vi "FieldDisplaySmall_OLD.vi"() -> ()   [LabVIEW 2025]
uses:
  <vilib>/Rock Robotics/WPI/ThirdParty/JAS_Junk/TrajLib/TypeDef/FieldDisp_ElementPicture.ctl
  <vilib>/Rock Robotics/WPI/ThirdParty/JAS_Junk/TrajLib/Rotation2d_CreateAngle.vi
  <vilib>/Rock Robotics/WPI/ThirdParty/JAS_Junk/TrajLib/Translation2d_Create.vi
  <vilib>/Rock Robotics/WPI/ThirdParty/JAS_Junk/TrajLib/VI/FieldDisp_Element_Rotate.vi
  <vilib>/Rock Robotics/WPI/ThirdParty/JAS_Junk/TrajLib/Conv_Meters_Inches.vi
  <vilib>/Rock Robotics/WPI/ThirdParty/JAS_Junk/TrajLib/Conv_Radians_Deg.vi
  <vilib>/picture/pixmap.llb/Flatten Pixmap.vi
  <vilib>/picture/pictutil.llb/Create Mask.vi
  <vilib>/picture/picture.llb/Draw Flattened Pixmap.vi
  <vilib>/Rock Robotics/WPI/ThirdParty/JAS_Junk/TrajLib/Trajectory_Library.lvlib
panel:
  out "Rear Side Last Sec Cnt":i32 format="%10.0f"
  out "Rear Back Last Sec Cnt":i32 format="%10.0f"
  out "Right Last Sec Cnt":i32 format="%10.0f"
  out "Left Last Sec Cnt":i32 format="%10.0f"
  out "ROBOT 2":T1
  out "Rear Side Tag Found":bool
  out "Rear Side Cam Conn":bool
  out "Rear Back Tag Found":bool
  out "Rear Back Cam Conn":bool
  out "Driver Orient Deg":dbl format="%11.1f"
  out "Driver Y Ft":dbl format="%11.2f"
  out "Driver X Ft":dbl format="%11.2f"
  out "ROBOT":T1
  out "Robot Orient Deg":dbl format="%11.1f"
  out "Robot Y Ft":dbl format="%11.2f"
  out "Robot X Ft":dbl format="%11.2f"
  out "Right April Tag Found":bool
  out "Left April Tag Found":bool
  out "Right Cam Connected":bool
  out "Left Cam Connected":bool
  out "Field Picture":picture
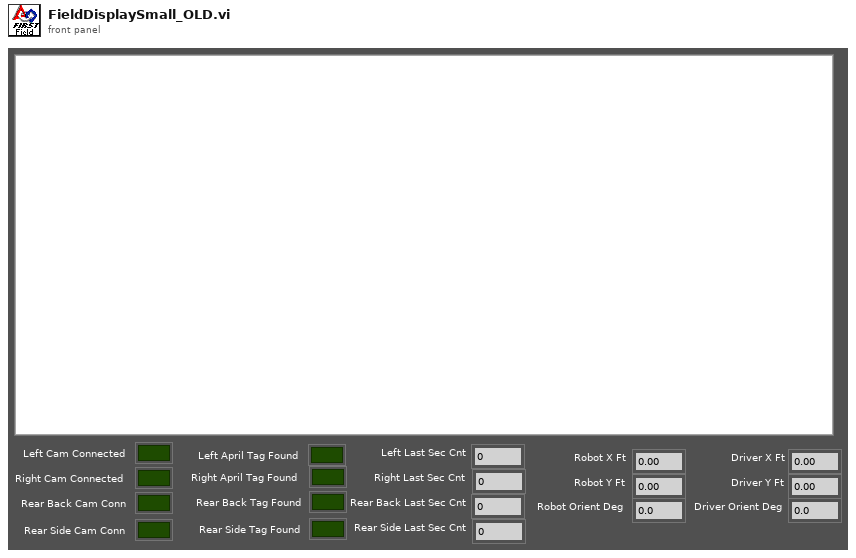
[diagram p1: front panel]
types:
  T1 = typedef "Trajectory_Library.lvlib/FieldDisp_ElementPicture.ctl" = picture
  T2 = typedef "Trajectory_Library.lvlib/FieldDisp_FieldElement.ctl" = cluster{"ONE-8-bit pixmap":u8[][], "Two-Array":cdb[][], "Three-Numeric":i32, "Four-Numeric":i32, "Five-Numeric":cdb, "Six-colors":u32[], "Seven-new element/subarray":u32, "Left Pixel":dbl, "Top Pixel":dbl, "Width Pix/Ft":dbl, "Height Pix/Ft":dbl, "Element Picture Ref":refnum<vi>}
  T3 = typedef "Trajectory_Library.lvlib/POSE2D.ctl" = cluster{"TRANSLATION":T4, "ROTATION":T5}
  T4 = typedef "Trajectory_Library.lvlib/TRANSLATION2D.ctl" = cluster{"X":dbl, "Y":dbl}
  T5 = typedef "Trajectory_Library.lvlib/ROTATION2D.ctl" = cluster{"VALUE":dbl, "COS":dbl, "SIN":dbl}
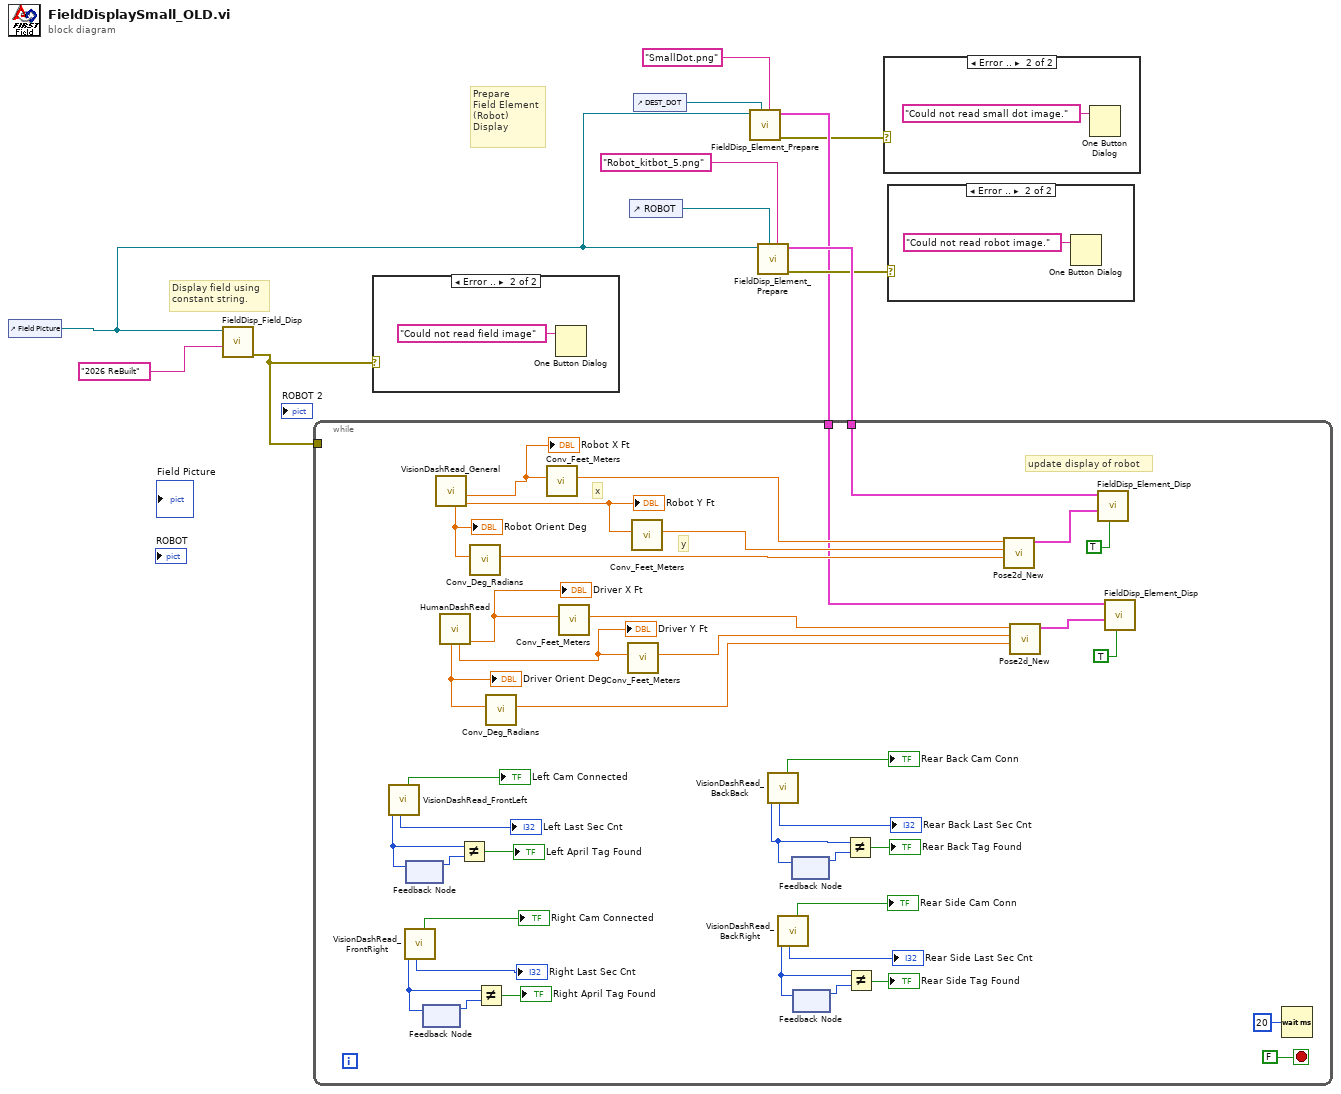
[diagram p0: block diagram]
diagram:
  # "Prepare\nField Element\n(Robot)\nDisplay"
  # "Display field using\nconstant string."
  n1 = control-ref of="Field Picture"() -> (w3:refnum<vi>)
  n2 = call <vilib>:"FieldDisp_Field_Disp.vi"("Field Selector"="2026 ReBuilt", "Picture in"=w3) -> ("error out"=w6:errorcluster)  [unwired: 9 in]
  n3 = case shown="Error .." w6 {
    frame No Error {
    }
    frame Error {
      n4 = One Button Dialog(message="Could not read field image") -> ()  [unwired: 1 in, 1 out]
    }
  }
  n5 = control-ref of="ROBOT"() -> (w9:refnum<vi>)
  n6 = control-ref of="DEST_DOT"() -> (w5:refnum<vi>)
  n7 = call <vilib>:"FieldDisp_Element_Prepare.vi"("Element File Name"="SmallDot.png" ("Picture FIle Name"), "Element Picture Ref"=w5, "Field Picture Ref"=w3) -> ("error out"=w1:errorcluster, "Field Element Info"=w2:T2)  [unwired: 7 in]
  n8 = call <vilib>:"FieldDisp_Element_Prepare.vi"("Element File Name"="Robot_kitbot_5.png" ("Picture FIle Name"), "Element Picture Ref"=w9, "Field Picture Ref"=w3) -> ("error out"=w7:errorcluster, "Field Element Info"=w8:T2)  [unwired: 7 in]
  n9 = while {
    tunnel: w8 -> [w51]
    tunnel: w6 -> [_]
    tunnel: w2 -> [w26]
    stop <- FALSE stop-if-true
    # "update display of robot"
    # "y"
    # "x"
    n10 = call "VisionDashRead_FrontLeft.vi"() -> ("FL Conn"=→"Left Cam Connected":bool, "FL Last Sec Cnt"=→"Left Last Sec Cnt":i64, "FL Count"=w36:i64)  [unwired: 2 in, 7 out]
    n11 = call "VisionDashRead_FrontRight.vi"() -> ("FR Conn"=→"Right Cam Connected":bool, "FR Last Sec Cnt"=→"Right Last Sec Cnt":i64, "FR Count"=w34:i64)  [unwired: 2 in, 7 out]
    n12 = feedback #1() -> (w47:i64)  [unwired: 1 in]
    n13 = feedback-in #1(w36) -> ()
    n14 = feedback #2() -> (w46:i64)  [unwired: 1 in]
    n15 = feedback-in #2(w34) -> ()
    n16 = call "VisionDashRead_General.vi"() -> ("PosYFt"=w39:dbl, "PosXFt"=w40:dbl, "PosOrientDeg"=w38:dbl)  [unwired: 4 in, 5 out]
    "Robot X Ft" <- w40
    "Robot Y Ft" <- w39
    "Robot Orient Deg" <- w38
    n17 = call "HumanDashRead.vi"() -> ("TrajDestX_Ft"=w24:dbl, "TrajDestY_Ft"=w22:dbl, "TrajDestAng_Deg"=w20:dbl)  [unwired: 5 in, 4 out]
    "Driver X Ft" <- w24
    "Driver Y Ft" <- w22
    "Driver Orient Deg" <- w20
    n18 = Not Equal?(x=w36, y=w47) -> (x != y?=→"Left April Tag Found":bool)
    n19 = call <vilib>:"Conv_Deg_Radians.vi"("Degress"=w38) -> ("Radians"=w48:dbl)  [unwired: 10 in]
    n20 = Not Equal?(x=w34, y=w46) -> (x != y?=→"Right April Tag Found":bool)
    n21 = call <vilib>:"Conv_Deg_Radians.vi"("Degress"=w20) -> ("Radians"=w19:dbl)  [unwired: 10 in]
    n22 = call <vilib>:"Conv_Feet_Meters.vi"("Feet"=w40) -> ("Meters"=w50:dbl)  [unwired: 10 in]
    n23 = call <vilib>:"Conv_Feet_Meters.vi"("Feet"=w24) -> ("Meters"=w23:dbl)  [unwired: 10 in]
    n24 = call <vilib>:"Conv_Feet_Meters.vi"("Feet"=w22) -> ("Meters"=w21:dbl)  [unwired: 10 in]
    n25 = call <vilib>:"Conv_Feet_Meters.vi"("Feet"=w39) -> ("Meters"=w49:dbl)  [unwired: 10 in]
    n26 = call "VisionDashRead_BackBack.vi"() -> ("BB Conn"=→"Rear Back Cam Conn":bool, "BB Last Sec Cnt"=→"Rear Back Last Sec Cnt":i64, "BB Count"=w29:i64)  [unwired: 2 in, 7 out]
    n27 = call "VisionDashRead_BackRight.vi"() -> ("BR Conn"=→"Rear Side Cam Conn":bool, "BR Last Sec Cnt"=→"Rear Side Last Sec Cnt":i64, "BR Count"=w30:i64)  [unwired: 2 in, 7 out]
    n28 = feedback #3() -> (w32:i64)  [unwired: 1 in]
    n29 = feedback-in #3(w29) -> ()
    n30 = feedback #4() -> (w31:i64)  [unwired: 1 in]
    n31 = feedback-in #4(w30) -> ()
    n32 = Not Equal?(x=w29, y=w32) -> (x != y?=→"Rear Back Tag Found":bool)
    n33 = Not Equal?(x=w30, y=w31) -> (x != y?=→"Rear Side Tag Found":bool)
    n34 = call <vilib>:"Pose2d_New.vi"("Heading"=w48, "Y"=w49, "X"=w50) -> ("out POSe"=w43:T3)  [unwired: 8 in]
    n35 = call <vilib>:"Pose2d_New.vi"("Heading"=w19, "Y"=w21, "X"=w23) -> ("out POSe"=w25:T3)  [unwired: 8 in]
    n36 = call <vilib>:"FieldDisp_Element_Disp.vi"("Visible"=TRUE, "Element Pose"=w43, "Element Info"=w51) -> ()  [unwired: 9 in]
    n37 = call <vilib>:"FieldDisp_Element_Disp.vi"("Visible"=TRUE, "Element Pose"=w25, "Element Info"=w26) -> ()  [unwired: 9 in]
    n38 = Wait (ms)(milliseconds to wait=u32 20) -> ()  [unwired: 1 out]
  }
  n39 = case shown="Error .." w1 {
    frame No Error {
    }
    frame Error {
      n40 = One Button Dialog(message="Could not read small dot image.") -> ()  [unwired: 1 in, 1 out]
    }
  }
  n41 = case shown="Error .." w7 {
    frame No Error {
    }
    frame Error {
      n42 = One Button Dialog(message="Could not read robot image.") -> ()  [unwired: 1 in, 1 out]
    }
  }
